vi "DAQmx Wait Until Done.vi"(0 "task/channels in":refnum<k21>, 7 "timeout (sec)":dbl=10.0 format="%0.2f", 11 "error in":errorcluster) -> (4 "task out":refnum<k21>, 15 "error out":errorcluster)   [LabVIEW 2013]
doc: "Waits for the measurement or generation to complete. Use this VI to ensure that the specified operation is complete before you stop the task."
uses:
  nilvaiu.dll
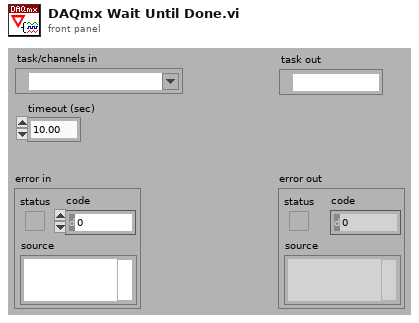
[diagram p1: front panel]
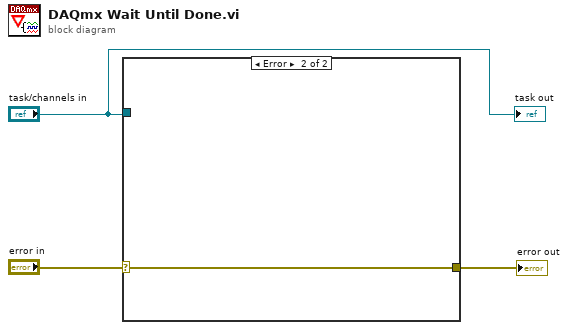
[diagram p0: block diagram]
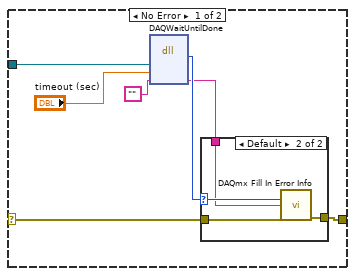
[diagram p2: hidden frame]
diagram:
  n1 = case shown="Error" "error in" {
    selector: "error in" -> [w6 w16]
    tunnel: [w8 w16] -> w1
    tunnel: "task/channels in" -> [w10 _]
    frame No Error {
      n2 = dll-call lib="nilvaiu.*" fn="DAQWaitUntilDone"("taskID"=w10, "timeout"="timeout (sec)", "extendedErrorInfo"="") -> (w9:i32, "extendedErrorInfo"=w5:string)  [unwired: 4 in, 3 out]
      n3 = case shown="Default" w9 {
        selector: w9 -> [_ w14]
        tunnel: [w11 w15] -> w8
        tunnel: w5 -> [_ w13]
        tunnel: w6 -> [w11 w12]
        frame 0 {
        }
        frame Default {
          n4 = call "DAQmx Fill In Error Info.vi"("status code"=w14, "extended error info"=w13, "error in"=w12) -> ("error out"=w15:errorcluster)  [unwired: 1 in, 11 out]
        }
      }
    }
    frame Error {
    }
  }
  "error out" <- w1
  "task out" <- "task/channels in"
